vi "Write Request time.vi"(8 "error in (no error)":errorcluster, 10 "Request time":timestamp, 11 "Recieve Request for Result Msg in":refnum<class "Recieve Request for Result Msg.lvclass">) -> (0 "error out":errorcluster, 3 "Recieve Request for Result Msg out":refnum<class "Recieve Request for Result Msg.lvclass">)   [LabVIEW 2015, in "Recieve Request for Result Msg.lvclass"]
uses:
  Recieve Request for Result Msg.lvclass
  Recieve Request for Result Msg.lvclass/Recieve Request for Result Msg.ctl
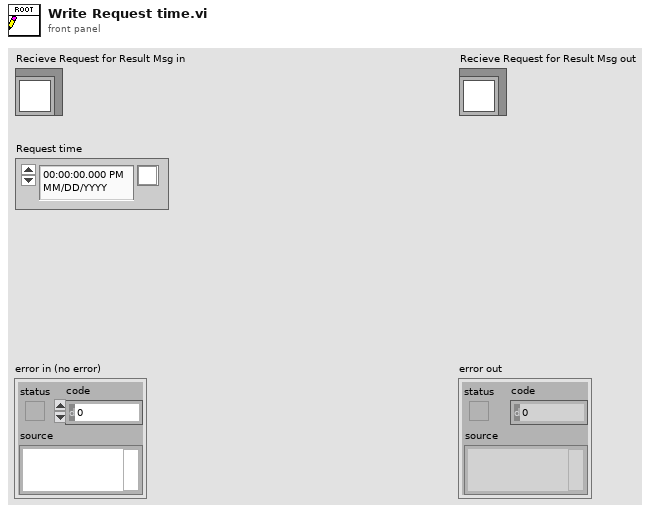
[diagram p1: front panel]
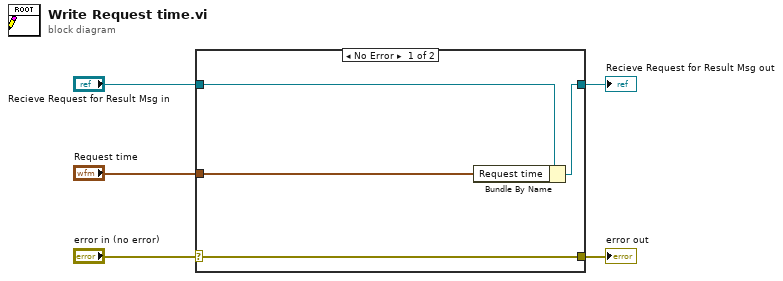
[diagram p0: block diagram]
diagram:
  n1 = case shown="No Error" "error in (no error)" {
    selector: "error in (no error)" -> [w9 w10]
    tunnel: [w9 w10] -> w4
    tunnel: [w7 w11] -> w2
    tunnel: "Recieve Request for Result Msg in" -> [w8 w11]
    tunnel: "Request time" -> [w6 _]
    frame No Error {
      n2 = Bundle By Name(cluster=w8, "Request time"=w6) -> (w7:refnum<class "Recieve Request for Result Msg.lvclass">)
    }
    frame Error {
    }
  }
  "error out" <- w4
  "Recieve Request for Result Msg out" <- w2
